vi "单个流程写入.vi"(5 "简易流程Id":u16(ring), 6 "是否是简易流程":bool, 7 "添加的路径":path, 8 "error in (no error)":errorcluster caption="错误输入（无错误）", 9 "量程":enum16{"低量程", "高量程"}(ring), 10 "测量模式":T1(ring), 11 "测量参数":u16(ring) items=["总氮"=2, "总磷"=1, "氨氮"=3, "COD"=22]) -> (0 "error out":errorcluster caption="错误输出", 3 "大小":i32)   [LabVIEW 2016, in "斯坦道CODcr.lvlib"]
uses:
  <vilib>/Plasmionique/MB Master/MB Master.lvlib
panel:
  out "流程写入进度":dbl
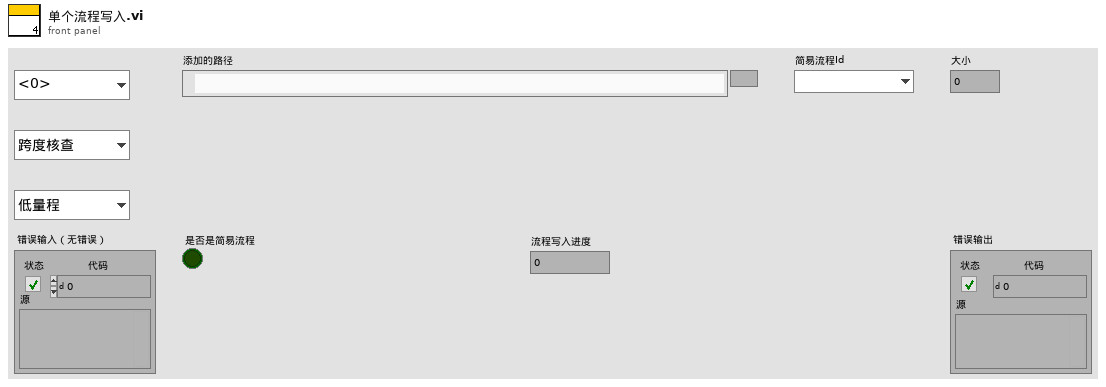
[diagram p1: front panel]
types:
  T1 = enum16{"跨度核查", "水样测量", "零点核查", "标样核查", "加标回收", "快捷测试", "空白校准", "标样校准"}
  T2 = cluster{"测量参数":u16, "测量模式":enum16{"跨度核查", "水样测量", "零点核查", "标样核查", "加标回收", "快捷测试", "空白校准", "标样校准"}, "量程":enum16{"低量程", "高量程"}}
  T3 = cluster{"port":i32, "dac":u8, "adc":u8, "time":u16, "步骤名":string}[]
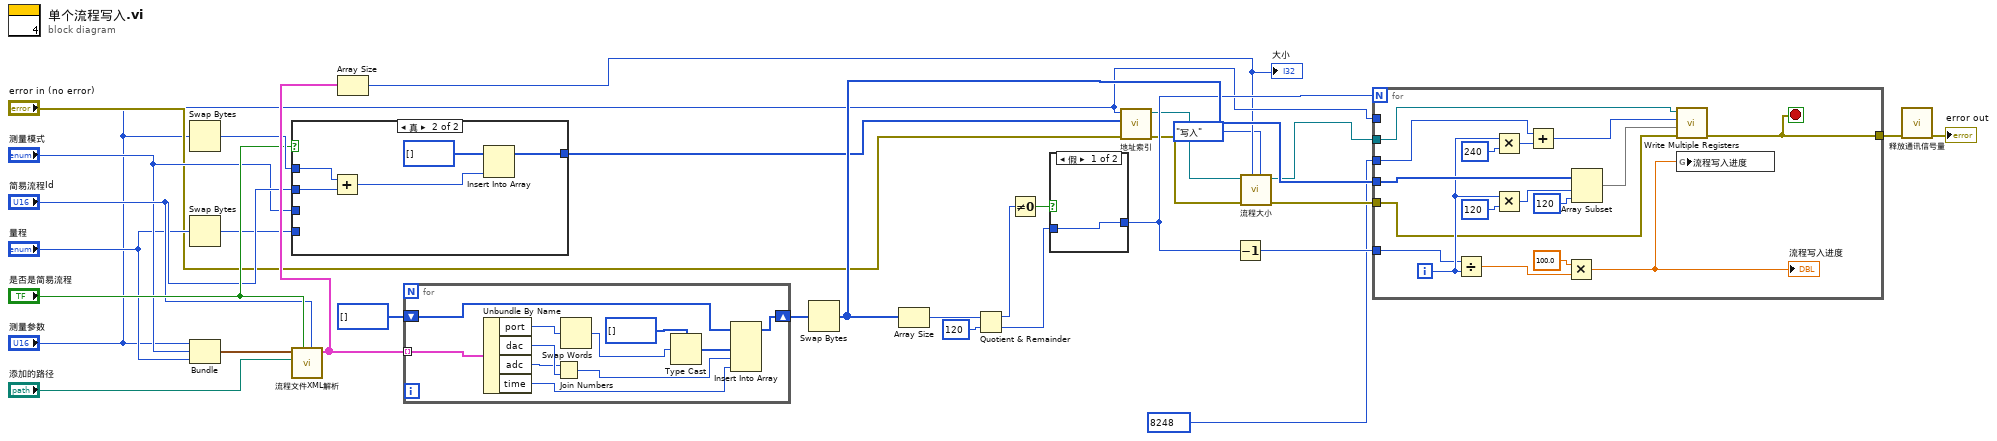
[diagram p0: block diagram]
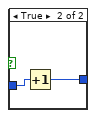
[diagram p2: hidden frame]
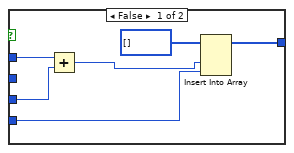
[diagram p3: hidden frame]
diagram:
  n1 = Swap Bytes(anything="测量参数") -> (byte swapped=w26:u16)
  n2 = Swap Bytes(anything="量程") -> (byte swapped=w22:u16)
  n3 = Bundle("测量参数"="测量参数", "测量模式"="测量模式", "量程"="量程") -> (w31:T2)  [unwired: 1 in]
  n4 = case shown="真" "是否是简易流程" {
    tunnel: [w35 w40] -> w12
    tunnel: "测量模式" -> [w34 _]
    tunnel: w26 -> [w33 w39]
    tunnel: w22 -> [w32 _]
    tunnel: "简易流程Id" -> [_ w38]
    frame False {
      n5 = Add(x=w33, y=w34) -> (x+y=w37:u16)
      n6 = Insert Into Array(array=u16[] [] ("数组"), new element #1=w37, new element #2=w32) -> (w35:u16[])  [unwired: 1 in]
    }
    frame True {
      n7 = Add(x=w39, y=w38) -> (x+y=w42:u16)
      n8 = Insert Into Array(array=u16[] [] ("数组"), new element=w42) -> (w40:u16[])  [unwired: 1 in]
    }
  }
  n9 = call "流程文件XML解析.vi"("简易流程Id"="简易流程Id", "是否是简易流程"="是否是简易流程", "添加的路径"="添加的路径", "参数簇"=w31) -> ("数组"=w27:T3)  [unwired: 7 in]
  n10 = Array Size(array=w27) -> (size(s)=w7:i32)
  "大小" <- w7
  n11 = for {
    tunnel: w27 -> [w53] mode=indexing
    shift-right: [w48] -> w28
    shift-left: u16[] [] -> [w46]
    n12 = Unbundle By Name(w53) -> ("port"=w51:i32, "dac"=w44:u8, "adc"=w43:u8, "time"=w49:u16)
    n13 = Join Numbers(hi=w43, lo=w44) -> ((hi.lo)=w50:u16)
    n14 = Swap Words(1:w51) -> (0:w45:i32)
    n15 = Type Cast(type=u16[] [], x=w45) -> (*(type *) &x=w47:u16[])
    n16 = Insert Into Array(array=w46, new element #1=w47, new element #2=w50, new element #3=w49) -> (w48:u16[])  [unwired: 1 in]
  }
  n17 = Swap Bytes(anything=w28) -> (byte swapped=w20:u16[])
  n18 = Array Size(array=w20) -> (size(s)=w19:i32)
  n19 = Quotient & Remainder(x=w19, y=120) -> (x-y*floor(x/y)=w17:i32, floor(x/y)=w15:i32)
  n20 = Not Equal To 0?(x=w17) -> (x != 0?=w16:bool)
  n21 = case shown="假" w16 {
    tunnel: w15 -> [w54 w56]
    tunnel: [w54 w55] -> w14
    frame False {
    }
    frame True {
      n22 = Increment(x=w56) -> (x+1=w55:i32)
    }
  }
  n23 = call "地址索引.vi"("error in (no error)"="error in (no error)", "values"=w12, "测量参数"="测量参数") -> ("error out"=w9:errorcluster, "MB session out"=w8:refnum<class "MB_Master.lvclass">)  [unwired: 7 in]
  n24 = Decrement(x=w14) -> (x-1=w13:i32)
  n25 = call "流程大小.vi"("功能"=enum16{"写入", "读取"}."写入", "大小"=w7, "error in (no error)"=w9, "MB session in"=w8) -> ("error out"=w5:errorcluster, "MB session out"=w6:refnum<class "MB_Master.lvclass">)  [unwired: 5 in, 1 out]
  n26 = for {
    N: w14 -> [_]
    tunnel: u16 8248 ("starting address") -> [w73]
    tunnel: [w57] -> w4
    tunnel: w20 -> [w67]
    tunnel: "测量参数" -> [_]
    tunnel: w13 -> [w62]
    tunnel: w6 -> [w61]
    tunnel: w5 -> [w60]
    i -> [w65]
    stop <- w57 stop-if-true
    n27 = Divide(x=w62, y=w65) -> (x/y=w70:dbl)
    n28 = Multiply(x=w65, y=240) -> (x*y=w72:i32)
    n29 = Multiply(x=w65, y=120) -> (x*y=w64:i32)
    n30 = Add(x=w73, y=w72) -> (x+y=w59:i32)
    n31 = Multiply(x=100.0, y=w70) -> (x*y=w68:dbl)
    "流程写入进度" <- w68
    n32 = Array Subset(array=w67, index=w64, length=120 ("长度")) -> (w58:u16[])
    n33 = call <vilib>:"Write Multiple Registers.vi"("error in (no error)"=w60, "values"=w58, "starting address"=w59, "MB session in"=w61) -> ("error out"=w57:errorcluster)  [unwired: 6 in, 1 out]
    n34 = global write "VAR总磷总氮全局变量.vi" "流程写入进度"(w68) -> ()
  }
  n35 = call "释放通讯信号量.vi"("error in (no error)"=w4) -> ("error out"=→"error out":errorcluster)  [unwired: 10 in]
